vi "Initialize.vi"(8 "error in (no error)":errorcluster, 10 "Parameters in":refnum<class "Abstract Init Parameters.lvclass">[](array[class]), 11 "Abstract Producer in":refnum<class "Abstract Producer.lvclass">) -> (0 "error out":errorcluster, 3 "Abstract Producer out":refnum<class "Abstract Producer.lvclass">)   [LabVIEW 2027, in "Messaging.lvlib" / "Abstract Producer.lvclass"]
uses:
  Abstract Producer.lvclass
  Parameters/Abstract Init Parameters/Abstract Init Parameters.lvclass
  Consumer Information.ctl
  Message Queue/Abstract Message Queue/Abstract Message Queue.lvclass
  Abstract Producer.lvclass/Abstract Producer.ctl
  Messaging.lvlib
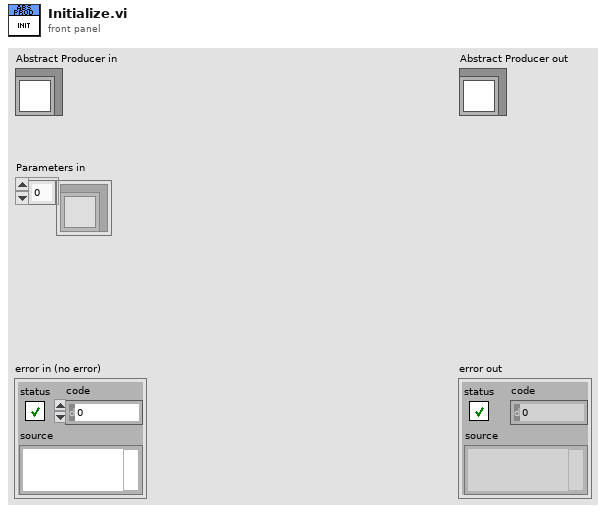
[diagram p1: front panel]
types:
  T1 = typedef "Messaging.lvlib/Abstract Producer.lvclass/Consumer Information.ctl" = cluster{"Name":string, "Request Queue":refnum<class "Abstract Message Queue.lvclass">, "Response Queue":refnum<class "Abstract Message Queue.lvclass">}
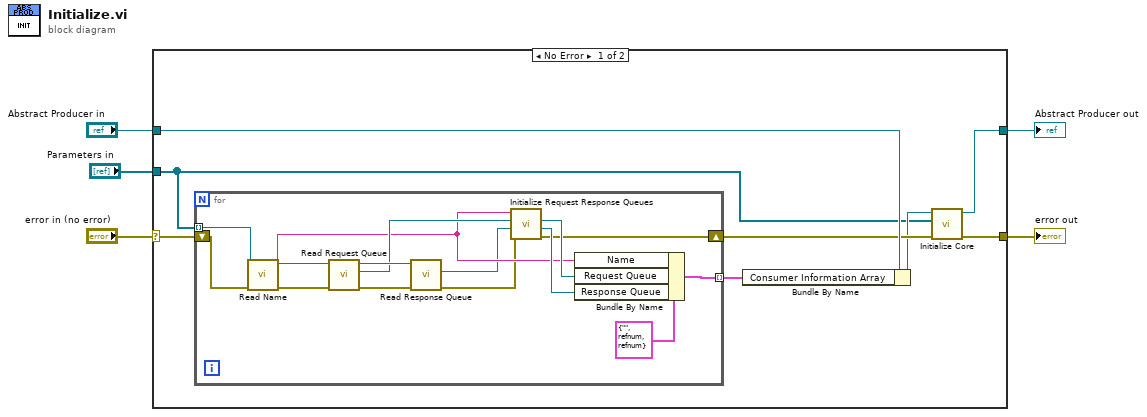
[diagram p0: block diagram]
diagram:
  n1 = case shown="No Error" "error in (no error)" {
    selector: "error in (no error)" -> [w13 w30]
    tunnel: [w9 w30] -> w4
    tunnel: [w7 w29] -> w2
    tunnel: "Abstract Producer in" -> [w11 w29]
    tunnel: "Parameters in" -> [w6 _]
    frame No Error {
      n2 = for {
        tunnel: w6 -> [w19] mode=indexing
        shift-right: [w24] -> w10
        shift-left: w13 -> [w18]
        tunnel: [w25] -> w12 mode=indexing
        n3 = call-dynamic "Read Name.vi"("error in (no error)"=w18, "Abstract Init Parameters in"=w19) -> ("error out"=w21:errorcluster, "Name"=w16:string, "Abstract Init Parameters out"=w23:refnum<class "Abstract Init Parameters.lvclass">)  [unwired: 7 in]
        n4 = call-dynamic "Read Request Queue.vi"("error in (no error)"=w21, "Abstract Init Parameters in"=w23) -> ("error out"=w20:errorcluster, "Message Queue Library.lvlib:Abstract Message Queue.lvclass"=w17:refnum<class "Abstract Message Queue.lvclass">, "Abstract Init Parameters out"=w22:refnum<class "Abstract Init Parameters.lvclass">)  [unwired: 7 in]
        n5 = call-dynamic "Read Response Queue.vi"("error in (no error)"=w20, "Abstract Init Parameters in"=w22) -> ("error out"=w15:errorcluster, "Message Queue Library.lvlib:Abstract Message Queue.lvclass"=w14:refnum<class "Abstract Message Queue.lvclass">)  [unwired: 7 in, 1 out]
        n6 = call "Initialize Request Response Queues.vi"("error in (no error)"=w15, "Response Queue in"=w14, "Request Queue in"=w17, "Name"=w16) -> ("error out"=w24:errorcluster, "Response Queue out"=w26:refnum<class "Abstract Message Queue.lvclass">, "Request Queue out"=w27:refnum<class "Abstract Message Queue.lvclass">)  [unwired: 5 in]
        n7 = Bundle By Name(cluster=T1 {"Name"="", "Request Queue"=refnum, "Response Queue"=refnum} ("Consumer Information"), "Name"=w16, "Request Queue"=w27, "Response Queue"=w26) -> (w25:T1)
      }
      n8 = Bundle By Name(cluster=w11, "Consumer Information Array"=w12) -> (w8:refnum<class "Abstract Producer.lvclass">)
      n9 = call-dynamic "Initialize Core.vi"("error in (no error)"=w10, "Parameters"=w6, "Abstract Producer in"=w8) -> ("error out"=w9:errorcluster, "Abstract Producer out"=w7:refnum<class "Abstract Producer.lvclass">)  [unwired: 7 in]
    }
    frame Error {
    }
  }
  "error out" <- w4
  "Abstract Producer out" <- w2
